vi "Determine Chart Num.vi"(8 "error in (no error)":errorcluster, 11 "HistorianCharting in":refnum<class "HistorianCharting.lvclass">) -> (0 "error out":errorcluster, 3 "HistorianCharting out":refnum<class "HistorianCharting.lvclass">)   [LabVIEW 2020, in "VolatusGUIElements.lvlib" / "HistorianCharting.lvclass"]
uses:
  HistorianCharting.lvclass
  C:/dev/lv20CE/relink/lv-volatus/VolatusGUI/GUI Element/GUI Element.lvclass
  VolatusGUI/GUI Element/GUI Element.lvclass/GUI Element.ctl
  HistorianCharting.lvclass/HistorianCharting.ctl
  VolatusGUI/GUI Element/GUI Element.lvclass
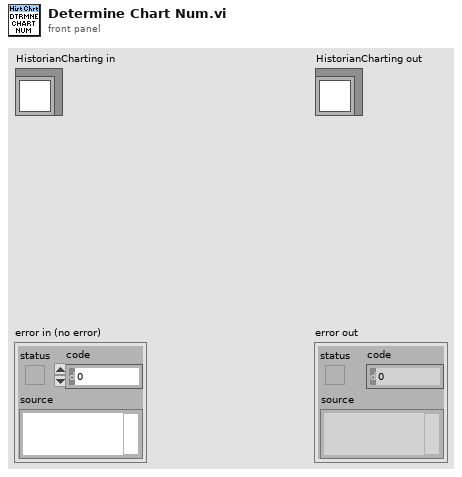
[diagram p1: front panel]
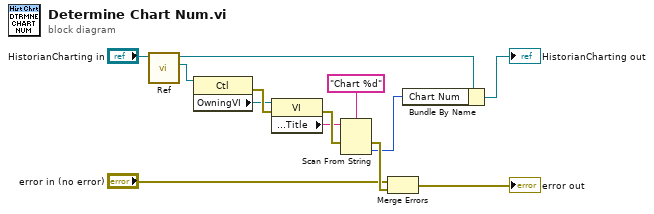
[diagram p0: block diagram]
diagram:
  n1 = call "Ref.vi"("GUI Element in"="HistorianCharting in") -> ("Ref"=w7:refnum<vi>, "GUI Element out"=w8:refnum<class "HistorianCharting.lvclass">)  [unwired: 9 in]
  n2 = property class="Ctl"(reference=w7) -> (error out=w11:errorcluster, "OwningVI"=w6:refnum<vi>)  [unwired: 1 in, 1 out]
  n3 = property class="VI"(reference=w6, error in=w11) -> (error out=w12:errorcluster, "Front Panel.Title"=w5:string)  [unwired: 1 out]
  n4 = Scan From String(format string="Chart %d", input string=w5, error in=w12) -> (error out=w13:errorcluster, output 1=w2:i32)  [unwired: 2 in, 2 out]
  n5 = Merge Errors("error in (no error)", w13) -> (→"error out":errorcluster)
  n6 = Bundle By Name(cluster=w8, "Chart Num"=w2) -> (→"HistorianCharting out":refnum<class "HistorianCharting.lvclass">)
